vi "Scale Data.vi"(9 "Data":dbl[][](array[numeric]), 11 "DataProcessor in":refnum<class "DataProcessor.lvclass">) -> (1 "Scaled Data":dbl[][](array[numeric]), 3 "DataProcessor out":refnum<class "DataProcessor.lvclass">)   [LabVIEW 2020, in "VolatusData.lvlib" / "DataProcessor.lvclass"]
uses:
  DataProcessor.lvclass
  DataProcessor.lvclass/DataProcessor.ctl
  Volatus/Scaling/Scaling.lvclass
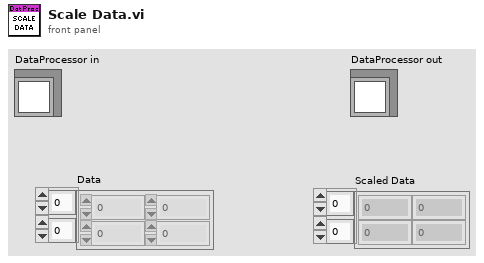
[diagram p1: front panel]
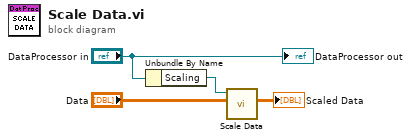
[diagram p0: block diagram]
diagram:
  n1 = Unbundle By Name("DataProcessor in") -> ("Scaling"=w3:refnum<class "Scaling.lvclass">)
  n2 = call "Scale Data.vi"("Data"="Data", "VolatusScaling in"=w3) -> ("Scaled Data"=→"Scaled Data":dbl[][])  [unwired: 8 in, 1 out]
  "DataProcessor out" <- "DataProcessor in"
